vi "Write Free-throw percentage.vi"(8 "error in (no error)":errorcluster, 10 "Free-throw percentage":dbl, 11 "Basketball Player in":refnum<class "Basketball Player.lvclass">) -> (0 "error out":errorcluster, 3 "Basketball Player out":refnum<class "Basketball Player.lvclass">)   [LabVIEW 2019, in "Basketball Player.lvclass"]
uses:
  Basketball Player.lvclass
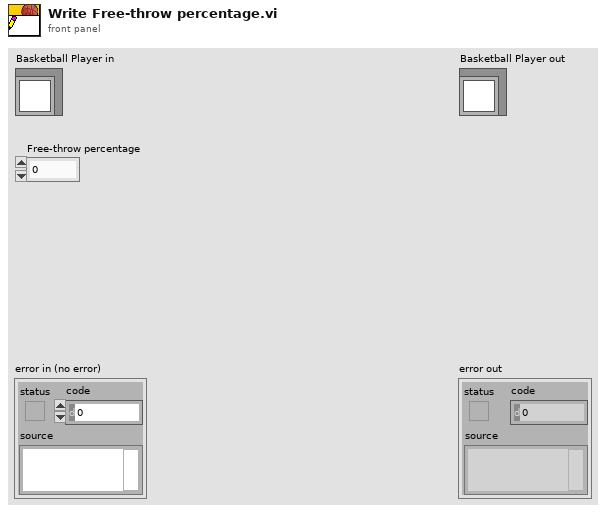
[diagram p1: front panel]
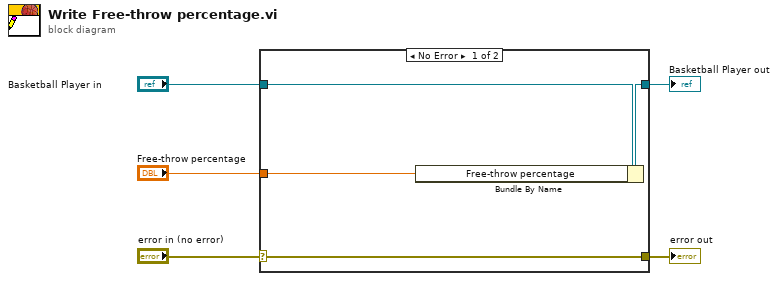
[diagram p0: block diagram]
diagram:
  n1 = case shown="No Error" "error in (no error)" {
    selector: "error in (no error)" -> [w9 w10]
    tunnel: [w9 w10] -> w4
    tunnel: [w7 w11] -> w2
    tunnel: "Basketball Player in" -> [w8 w11]
    tunnel: "Free-throw percentage" -> [w6 _]
    frame No Error {
      n2 = Bundle By Name(cluster=w8, "Free-throw percentage"=w6) -> (w7:refnum<class "Basketball Player.lvclass">)
    }
    frame Error {
    }
  }
  "error out" <- w4
  "Basketball Player out" <- w2
